vi "add timestamp to name.vi"(8 "error in (no error)":errorcluster, 11 "name":string) -> (0 "error out":errorcluster, 3 "build spec name":string)   [LabVIEW 2024, in "Builder.lvclass"]
uses:
  Builder.lvclass
  Builder.lvclass/Builder.ctl
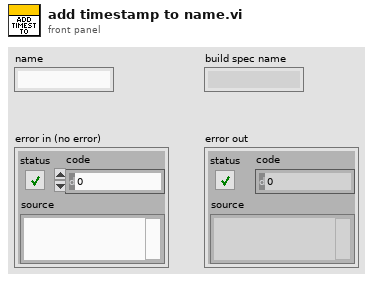
[diagram p1: front panel]
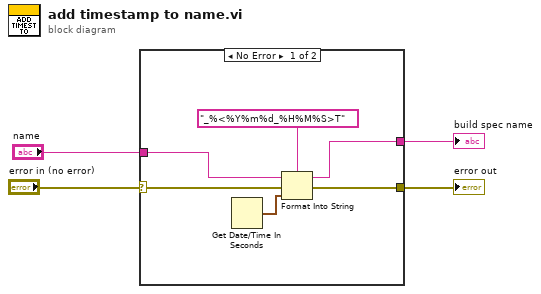
[diagram p0: block diagram]
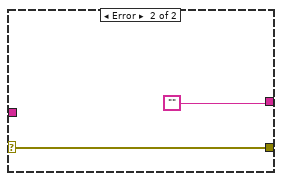
[diagram p2: hidden frame]
diagram:
  n1 = case shown="No Error" "error in (no error)" {
    selector: "error in (no error)" -> [w5 w12]
    tunnel: [w8 ""] -> w4
    tunnel: [w7 w12] -> w3
    tunnel: "name" -> [w6 _]
    frame No Error {
      n2 = Get Date/Time In Seconds() -> (seconds since 1Jan1904=w9:timestamp)
      n3 = Format Into String(format string="_%<%Y%m%d_%H%M%S>T", initial string=w6, error in=w5, w9) -> (resulting string=w8:string, error out=w7:errorcluster)
    }
    frame Error {
    }
  }
  "build spec name" <- w4
  "error out" <- w3
